vi "Is_It_Zero(Empty)_Point(in_Frame).vi"(1 "Index of dot \ninside frame":i32, 2 "Column (Frame)":dbl[](array[numeric])) -> (0 "It's zero point":bool)   [LabVIEW 2013]
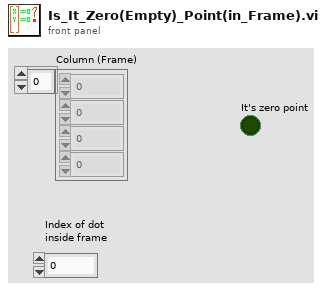
[diagram p1: front panel]
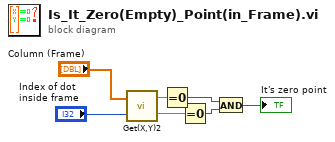
[diagram p0: block diagram]
diagram:
  n1 = call "Get(X,Y)2.vi"("[IN] index of (X,Y)"="Index of dot \ninside frame", "[IN] Array coordi\nnates (X,Y) in Frame"="Column (Frame)") -> ("[OUT] Y"=w5:dbl, "[OUT] X"=w6:dbl)
  n2 = Equal To 0?(x=w6) -> (x = 0?=w4:bool)
  n3 = Equal To 0?(x=w5) -> (x = 0?=w7:bool)
  n4 = And(x=w4, y=w7) -> (x .and. y?=→"It's zero point":bool)
